vi "parse and execute command.vi"(1 "Python Command":string) -> (0 "Python Return String":string)   [LabVIEW 2014]
panel:
  in  "base path":path
  out "error out":errorcluster
  in  "VI Refnum":refnum<vi>
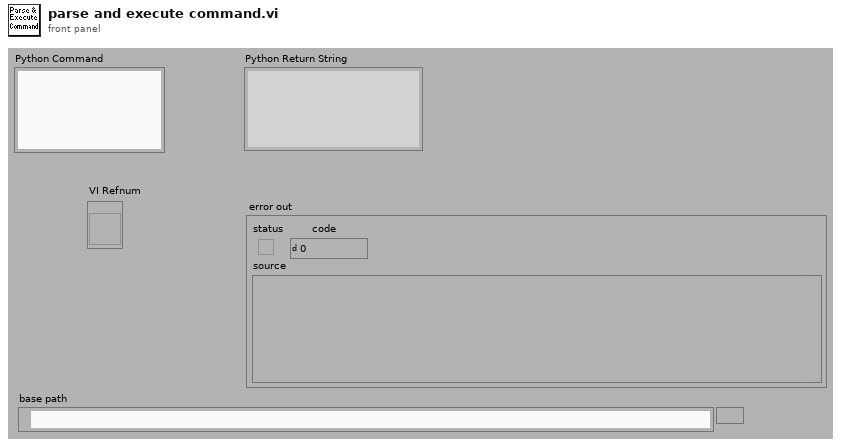
[diagram p1: front panel]
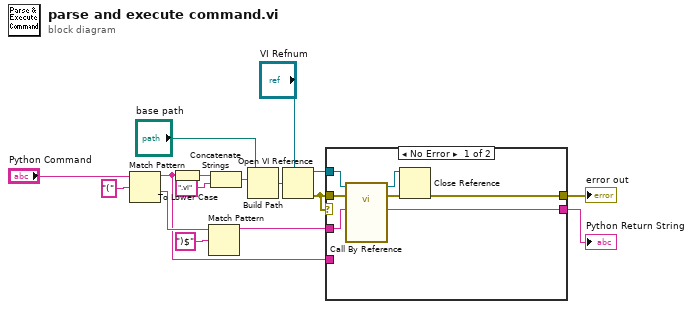
[diagram p0: block diagram]
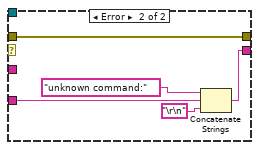
[diagram p2: hidden frame]
diagram:
  n1 = Match Pattern(string="Python Command", regular expression="(") -> (before substring=w5:string, after substring=w13:string)  [unwired: 1 in, 2 out]
  n2 = To Lower Case(string=w5) -> (all lower case string=w1:string)
  n3 = Match Pattern(string=w13, regular expression=")$") -> (before substring=w9:string)  [unwired: 1 in, 3 out]
  n4 = Concatenate Strings(w1, ".vi" ("regular expression")) -> (w3:string)
  n5 = Build Path(base path="base path", name or relative path=w3) -> (appended path=w4:path)
  n6 = Open VI Reference(type specifier VI Refnum (for type only)="VI Refnum", vi path=w4) -> (vi reference=w11:refnum<vi>, error out=w6:errorcluster)  [unwired: 4 in]
  n7 = case shown="No Error" w6 {
    tunnel: w11 -> [w23 _]
    tunnel: w6 -> [w21 w28]
    tunnel: [w19 w28] -> w10
    tunnel: w9 -> [w18 _]
    tunnel: [w17 w24] -> w8
    tunnel: w5 -> [_ w27]
    frame No Error {
      n8 = call-by-ref "?"(reference=w23, error in=w21, "Input"=w18) -> (reference out=w22:refnum<vi>, error out=w20:errorcluster, "Output"=w17:string)  [unwired: 9 in, 1 out]
      n9 = Close Reference(reference=w22, error in (no error)=w20) -> (error out=w19:errorcluster)
    }
    frame Error {
      n10 = Concatenate Strings("unknown command:" ("Output"), w27, "\r\n") -> (w24:string)
    }
  }
  "Python Return String" <- w8
  "error out" <- w10
